vi "ProdaNG.ProcessStepResult.Get.vi"(8 "error in (no error)":errorcluster, 9 "processStepId":i32, 10 "processResultId":string, 11 "dbHandle":i32) -> (0 "error out":errorcluster, 1 "Found":bool, 2 "ProcessStepResult":T1, 3 "dbHandle out":i32)   [LabVIEW 2016]
doc: "This function returns a ProcessStepResult structure for a process result and a process step. \nParameter:\nhandle is an Integer, which is returned by the function Login() at the creation of a new connection.\nprocessResultId is the Id of the associated process result.\nprocessStepId is the Id of the associated process step.\nprocessStepResult is a pointer on a ProcessStepResult structure, which is filled if the returncode is 0. The structure must be defined in the calling program.\nReturncodes:\n0 No error\n< 0 ORACLE Error code\n6 (ERROR_INVALID_HANDLE) in case of an invalid handle\n1403 Record does not exist"
uses:
  Controls/ProdaNG.ProcessStepResult.ctl
  Controls/ProdaNG.ProcessStepResultSize.ctl
  prodllNG.dll
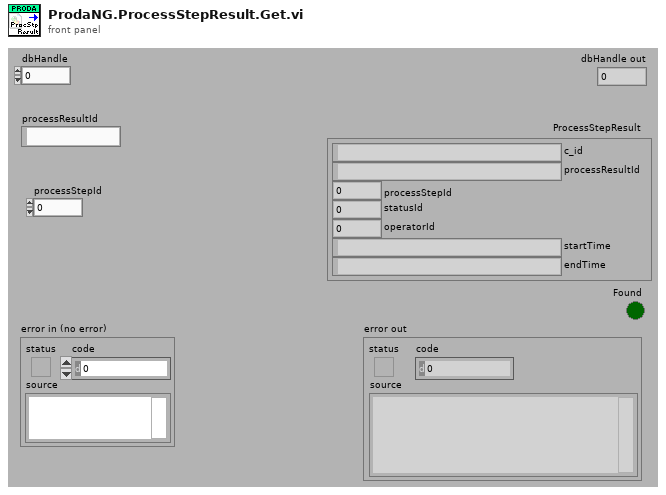
[diagram p1: front panel]
types:
  T1 = typedef "ProdaNG.ProcessStepResult.ctl" = cluster{"c_id":string, "processResultId":string, "processStepId":i32, "statusId":i32, "operatorId":i32, "startTime":string, "endTime":string}
  T2 = typedef "ProdaNG.ProcessStepResultSize.ctl" = cluster{"c_id":i32, "processResultId":i32, "processStepId":i32, "statusId":i32, "operatorId":i32, "startTime":i32, "endTime":i32}
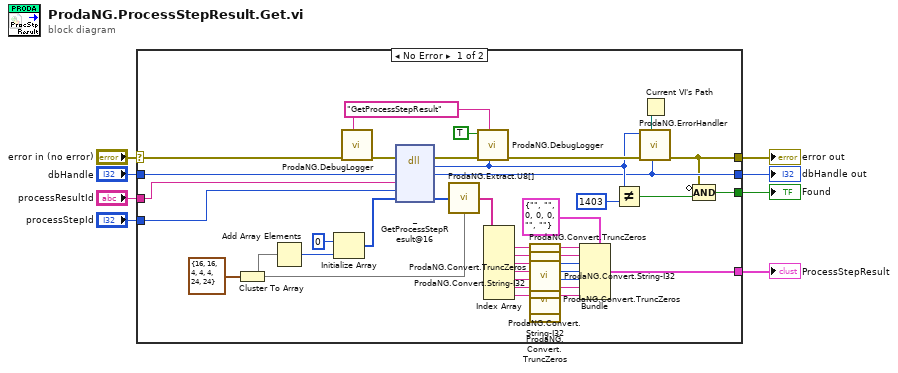
[diagram p0: block diagram]
diagram:
  n1 = case shown="No Error" "error in (no error)" {
    selector: "error in (no error)" -> [w24 w49]
    tunnel: [w9 w49] -> w7
    tunnel: "dbHandle" -> [w20 w48]
    tunnel: [w11 w48] -> w5
    tunnel: "processResultId" -> [w21 _]
    tunnel: "processStepId" -> [w19 _]
    tunnel: [w13 _] -> w2
    tunnel: [w10 _] -> w1
    frame No Error {
      w46 = "GetProcessStepResult" ("cmd")
      n2 = Cluster To Array(cluster=T2 {"c_id"=16, "processResultId"=16, "processStepId"=4, "statusId"=4, "operatorId"=4, "startTime"=24, "endTime"=24} ("ProcessStepResultSize")) -> (array=w37:i32[])
      n3 = Add Array Elements(numeric array=w37) -> (sum=w40:i32)
      n4 = Initialize Array(u8 0 ("element"), w40) -> (w36:u8[])
      n5 = call "ProdaNG.DebugLogger.vi"("cmd"=w46, "error in (no error)"=w24) -> ("error out"=w44:errorcluster)  [unwired: 9 in]
      n6 = dll-call lib="D:/svn/LineTraceSystem/SOFTWARE/sources/Database/ProdaNG/prodllNG.dll" fn="_GetProcessStepResult@16" ("ProDLL wrapper.dll:ProDLL_wrapper_GetWabcoParts_GetData")(error in=w44, "dbHandle"=w20, "productId"=w21, "processId"=w19, "processResult"=w36) -> (error out=w43:errorcluster, "return type"=w34:i32, "dbHandle"=w11:i32, "processResult"=w35:u8[])  [unwired: 4 in, 1 out]
      n7 = call "ProdaNG.Extract.U8[].vi"("unsigned byte array"=w35, "Sizes"=w37) -> ("Elements"=w39:string[])
      n8 = call "ProdaNG.DebugLogger.vi"("return type"=w34, "cmd"=w46, "error in (no error)"=w43, "done? (F)"=TRUE) -> ("error out"=w42:errorcluster)  [unwired: 7 in]
      n9 = Index Array(array=w39) -> (element #1=w26:string, element #2=w25:string, element #3=w33:string, element #4=w30:string, element #5=w15:string, element #6=w29:string, element #7=w18:string)  [unwired: 7 in]
      n10 = call "ProdaNG.Convert.TruncZeros.vi"("string with \\0s"=w26) -> ("LV string"=w28:string)  [unwired: 10 in]
      n11 = call "ProdaNG.Convert.TruncZeros.vi"("string with \\0s"=w25) -> ("LV string"=w27:string)  [unwired: 10 in]
      n12 = call "ProdaNG.Convert.String-I32.vi"("unsigned byte string"=w33) -> ("32bit integer"=w32:i32)  [unwired: 10 in]
      n13 = call "ProdaNG.Convert.String-I32.vi"("unsigned byte string"=w30) -> ("32bit integer"=w31:i32)  [unwired: 10 in]
      n14 = call "ProdaNG.Convert.String-I32.vi"("unsigned byte string"=w15) -> ("32bit integer"=w14:i32)  [unwired: 10 in]
      n15 = call "ProdaNG.Convert.TruncZeros.vi"("string with \\0s"=w29) -> ("LV string"=w16:string)  [unwired: 10 in]
      n16 = call "ProdaNG.Convert.TruncZeros.vi"("string with \\0s"=w18) -> ("LV string"=w17:string)  [unwired: 10 in]
      n17 = Bundle(cluster=T1 {"c_id"="", "processResultId"="", "processStepId"=0, "statusId"=0, "operatorId"=0, "startTime"="", "endTime"=""} ("ProcessStepResult"), "c_id"=w28, "processResultId"=w27, "processStepId"=w32, "statusId"=w31, "operatorId"=w14, "startTime"=w16, "endTime"=w17) -> (w13:T1)
      n18 = Not Equal?(x=w34, y=1403) -> (x != y?=w12:bool)
      n19 = Current VI's Path() -> (path=w47:path)
      n20 = call "ProdaNG.ErrorHandler.vi"("dbHandleIn"=w11, "Path"=w47, "error in"=w42, "output_parameter"=w34) -> ("error out"=w9:errorcluster)  [unwired: 7 in]
      n21 = Compound Arithmetic op=AND(invert w9, w12) -> (w10:bool)
    }
    frame Error {
    }
  }
  "error out" <- w7
  "dbHandle out" <- w5
  "ProcessStepResult" <- w2
  "Found" <- w1
